vi "RT Activated Task.vi"(7 "Enum":enum16{"Read", "Write"}(ring), 8 "error in (no error)":errorcluster, 9 "Start Time in":timestamp, 11 "Activate Task":T1={"Analog input"=TRUE, "Analog Output"=TRUE, "Digital input"=TRUE, "Digital output"=TRUE, "Thermocouple"=FALSE, "Strain Gauge"=TRUE, "Accelerometer"=TRUE}) -> (0 "error out":errorcluster, 1 "Start Time":timestamp, 2 "Activate Task 2":T1)   [LabVIEW 2022 SP3]
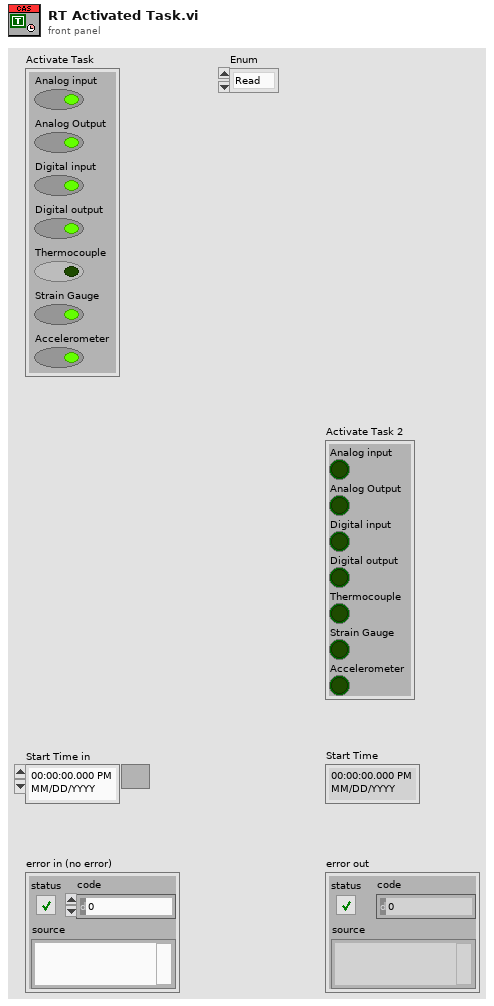
[diagram p1: front panel]
types:
  T1 = cluster{"Analog input":bool, "Analog Output":bool, "Digital input":bool, "Digital output":bool, "Thermocouple":bool, "Strain Gauge":bool, "Accelerometer":bool}
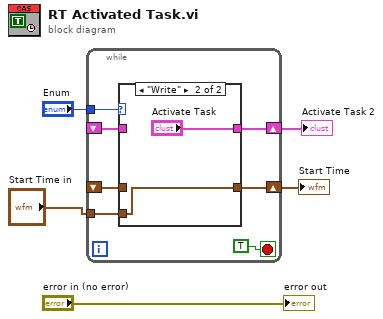
[diagram p0: block diagram]
diagram:
  n1 = while {
    tunnel: "Enum" -> [w12]
    shift-right: [w10] -> w2
    shift-left: _ -> [w9]
    shift-right: [w8] -> w3
    shift-left: _ -> [w7]
    tunnel: "Start Time in" -> [w6]
    stop <- TRUE stop-if-true
    n2 = case shown="\"Write\"" w12 {
      tunnel: [w14 w15] -> w10
      tunnel: w9 -> [w14 _]
      tunnel: [w13 "Activate Task"] -> w8
      tunnel: w7 -> [w13 _]
      tunnel: w6 -> [_ w15]
      frame "Read", Default {
      }
      frame "Write" {
      }
    }
  }
  "Start Time" <- w2
  "Activate Task 2" <- w3
  "error out" <- "error in (no error)"
